vi "Database Recordset Close.vi"(8 "error in (no error)":errorcluster caption="错误输入（无错误）", 11 "Database Recordset 输入":refnum<class "Database Recordset.lvclass"> caption="DNL_LabVIEW Object in") -> (0 "error out":errorcluster caption="错误输出", 3 "Database Connection输出":refnum<class "Database Connection.lvclass">)   [LabVIEW 2011, in "Database Recordset.lvclass"]
uses:
  Database Recordset.lvclass
  Connection/Database Connection.lvclass
  Database Recordset.lvclass/Database Recordset.ctl
panel:
  out "Database Recordset 输出":refnum<class "Database Recordset.lvclass"> caption="DNL_LabVIEW Object out"
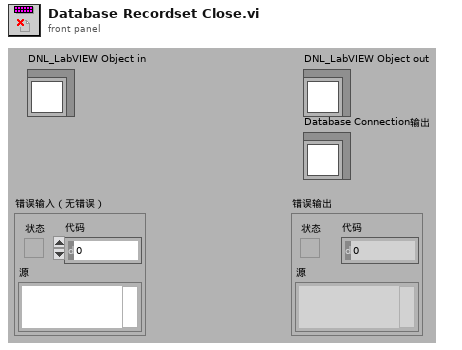
[diagram p1: front panel]
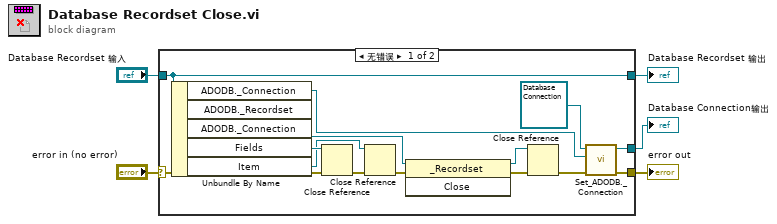
[diagram p0: block diagram]
diagram:
  n1 = case shown="无错误" "error in (no error)" {
    selector: "error in (no error)" -> [w10 w21]
    tunnel: [w12 w21] -> w4
    tunnel: [w19 w20] -> w2
    tunnel: "Database Recordset 输入" -> [w19 w20]
    tunnel: [w11 _] -> w1
    frame No Error {
      n2 = Unbundle By Name(w19) -> ("ADODB._Connection"=w14:refnum<k7>, "ADODB._Recordset"=w18:refnum<k7>, "Fields"=w9:refnum<k7>, "Item"=w6:refnum<k7>)  [unwired: 1 out]
      n3 = Close Reference(reference=w9, error in (no error)=w10) -> (error out=w8:errorcluster)
      n4 = Close Reference(reference=w6, error in (no error)=w8) -> (error out=w7:errorcluster)
      n5 = invoke class="_Recordset" method="Close"(reference=w18, error in=w7) -> (reference out=w17:refnum<k7>, error out=w16:errorcluster)  [unwired: 1 in, 1 out]
      n6 = Close Reference(reference=w17, error in (no error)=w16) -> (error out=w13:errorcluster)
      n7 = call "Set_ADODB._Connection.vi"("error in (no error)"=w13, "ADODB._Connection"=w14, "Database Connection输入"=refnum<class "Database Connection.lvclass"> refnum ("Database Connection.lvclass")) -> ("error out"=w12:errorcluster, "Database Connection输出"=w11:refnum<class "Database Connection.lvclass">)  [unwired: 7 in]
    }
    frame Error {
    }
  }
  "error out" <- w4
  "Database Recordset 输出" <- w2
  "Database Connection输出" <- w1
